vi "Get Set Init Parameters.vi"(8 "error in (no error)":errorcluster) -> (0 "error out":errorcluster)   [LabVIEW 2019, in "Spectrometer.lvlib"]
uses:
  Spectrometer.lvlib
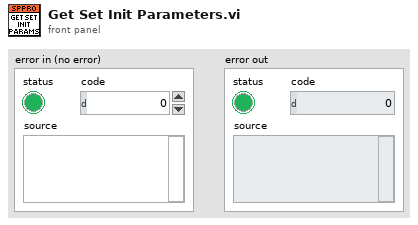
[diagram p1: front panel]
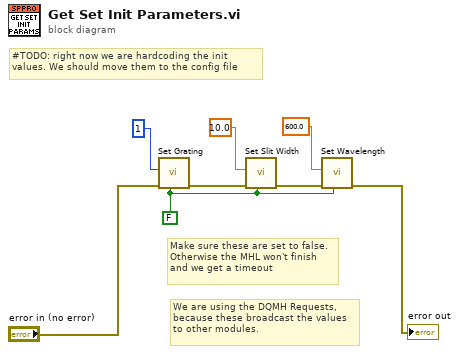
[diagram p0: block diagram]
diagram:
  w2 = FALSE ("wait for reply (T)")
  # "We are using the DQMH Requests,\nbecause these broadcast the values\nto other modules."
  # "Make sure these are set to false.\nOtherwise the MHL won't finish\nand we get a timeout"
  # "#TODO: right now we are hardcoding the init\nvalues. We should move them to the config file"
  n1 = call "Set Grating.vi"("wait for reply (T)"=w2, "error in (no error)"="error in (no error)", "Grating ID"=1) -> ("error out"=w8:errorcluster)  [unwired: 6 in, 2 out]
  n2 = call "Set Slit Width.vi"("wait for reply (T)"=w2, "error in (no error)"=w8, "Slit Width (um)"=10.0) -> ("error out"=w5:errorcluster)  [unwired: 6 in, 2 out]
  n3 = call "Set Wavelength.vi"("wait for reply (T)"=w2, "error in (no error)"=w5, "Wavelength"=600.0) -> ("error out"=→"error out":errorcluster)  [unwired: 6 in, 2 out]
